vi "Apply Configuration.vi"(8 "Error In":errorcluster, 11 "reference in":refnum<class "Instrument Base.lvclass">) -> (0 "Error Out":errorcluster, 3 "reference out":refnum<class "Instrument Base.lvclass">)   [LabVIEW 2023, in "HAL GOOP4.lvlib" / "Instrument Base.lvclass"]
uses:
  Instrument Base.lvclass
  Instrument Base.lvclass/Instrument Base.ctl
  Interfaces/IConfigure/IConfigure.lvclass
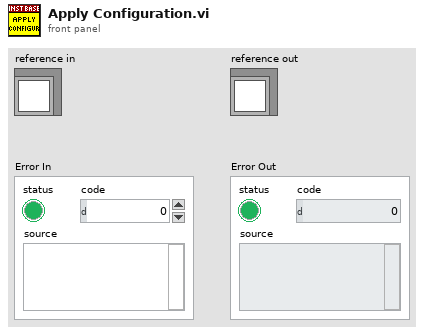
[diagram p1: front panel]
types:
  T1 = typedef "HAL GOOP4.lvlib/Instrument Base.lvclass/ObjectAttributes.ctl" = cluster{"Instr Identifier":string, "IConfigure":refnum<class "IConfigure.lvclass">}
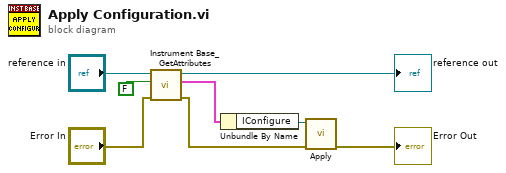
[diagram p0: block diagram]
diagram:
  n1 = call "Instrument Base_GetAttributes.vi"("Error In"="Error In", "OnlyGetDvrReference(False)"=FALSE, "reference in"="reference in") -> ("Error Out"=w4:errorcluster, "Data"=w1:T1, "reference out"=→"reference out":refnum<class "Instrument Base.lvclass">)  [unwired: 5 in, 1 out]
  n2 = Unbundle By Name(w1) -> ("IConfigure"=w2:refnum<class "IConfigure.lvclass">)
  n3 = call-dynamic "Apply.vi"("error in (no error)"=w4, "IConfigure in"=w2) -> ("error out"=→"Error Out":errorcluster)  [unwired: 8 in, 1 out]
